vi "应变测试.vi"(15 "stop":bool) -> ()   [LabVIEW 2010]
uses:
  Instance           1 16Saved   应变测试 .vi
  Instance           2 16Saved   应变测试 .vi
  <vilib>/Utility/TradDaqScaling.llb/Convert Strain Gauge Reading (scaler).vi
  <vilib>/Analysis/NI_AALBase.lvlib
panel:
  in  "激 励 电 压":dbl=5.0 format="%.3f"
  in  "应变片灵敏系数":dbl=2.0 format="%.2f"
  in  "置零":bool
  out "电压值\n   (mV)":dbl format="%.2f"
  out "最大挠度\n（mm)":dbl format="%.2f"
  out "电压值 \n   (mV)":dbl format="%.2f"
  out "应变 (με)":cluster{sgl, sgl}(graph)
  out "挠曲轴":cluster{i32[], dbl[]}(graph)
  # "应 变 测 试 实 验"
  # "全   桥"
  # "半   桥"
  # "全桥测试结果"
  # "半桥测试结果"
  # "时间（ms)"
  # "应变值\n（με）"
  # "应变值\n（με）"
  # "挠曲轴"
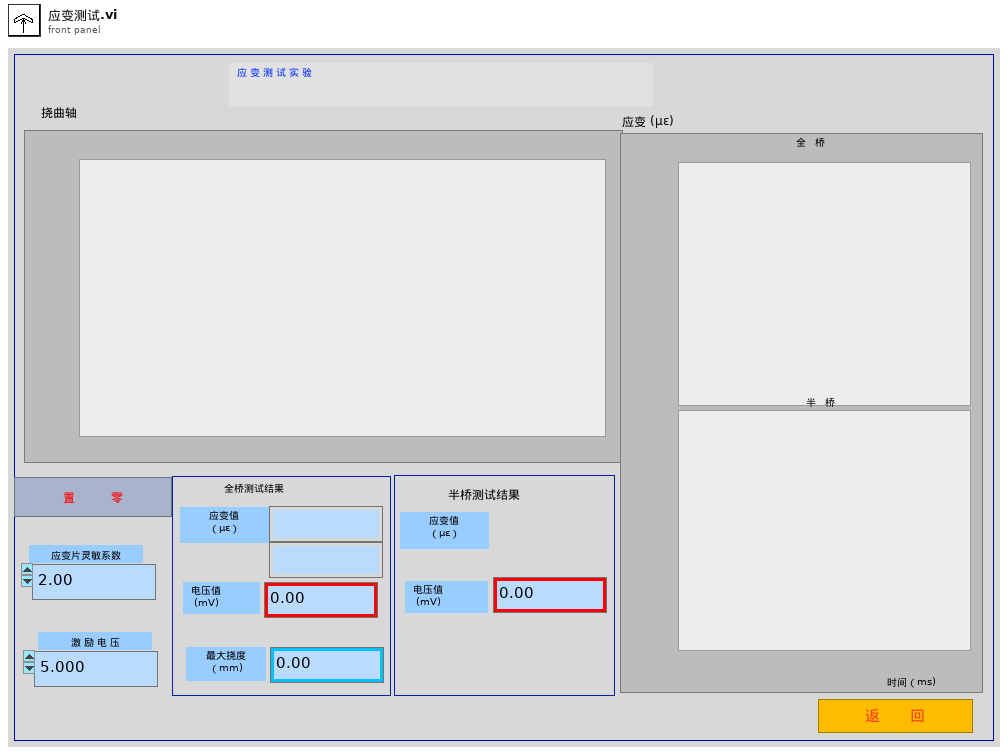
[diagram p1: front panel]
types:
  T1 = cluster{"梁的长度(mm)":dbl, "受力点距固定端(mm)":dbl, "应变片距固定端(mm)":dbl, "梁的厚度(mm)":dbl}
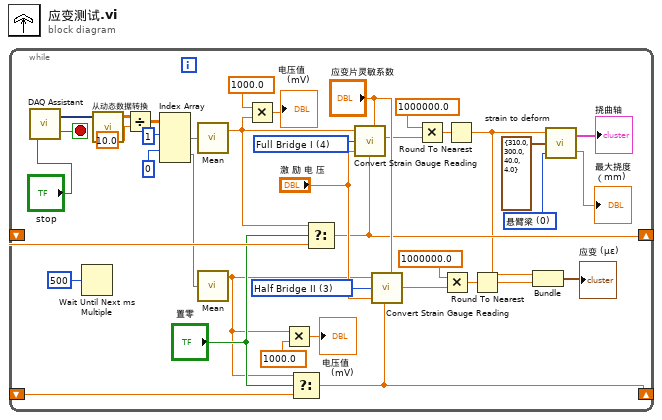
[diagram p0: block diagram]
diagram:
  n1 = while {
    shift-left: _ -> [w39]
    shift-right: [w16] -> _
    shift-right: [w24] -> _
    shift-left: _ -> [w25]
    stop <- w1 stop-if-true
    w9 = u16 0 items=["悬臂梁", "简支梁"] ("梁的结构")
    w34 = u16 3 items=["Qtr Bridge I", "Qtr Bridge II", "Half Bridge I", "Half Bridge II", "Full Bridge I", "Full Bridge II", "Full Bridge III"] ("Bridge Configuration\n(3:Half Bridge II)")
    w35 = u16 4 items=["Qtr Bridge I", "Qtr Bridge II", "Half Bridge I", "Half Bridge II", "Full Bridge I", "Full Bridge II", "Full Bridge III"] ("Bridge Configuration\n(3:Half Bridge II)")
    n2 = call "DAQ Assistant"("stop (F)"="stop") -> ("data"=w20:dynamicdata, "stopped"=w1:bool)  [unwired: 15 in, 2 out]
    n3 = Wait Until Next ms Multiple(millisecond multiple=u32 500 ("毫秒倍数")) -> ()  [unwired: 1 out]
    n4 = call "从动态数据转换"("Dynamic Data Type"=w20) -> ("Array"=w6:dbl[][])  [unwired: 3 in]
    n5 = Divide(x=w6, y=10.0) -> (x/y=w3:dbl[][])
    n6 = Index Array(array=w3, index (row) #1=1 ("disabled index (col)"), index (row) #2=0 ("index (col)")) -> (element #1=w5:dbl[], element #2=w4:dbl[])  [unwired: 2 in]
    n7 = call <vilib>:"Mean.vi"("X"=w5) -> ("mean"=w17:dbl)  [unwired: 1 out]
    n8 = call <vilib>:"Mean.vi"("X"=w4) -> ("mean"=w18:dbl)  [unwired: 1 out]
    n9 = Multiply(x=1000.0, y=w17) -> (x*y=→"电压值\n   (mV)":dbl)
    n10 = Multiply(x=w18, y=1000.0 ("x")) -> (x*y=→"电压值 \n   (mV)":dbl)
    n11 = Select(t=w18, s="置零", f=w25) -> (s? t:f=w24:dbl)
    n12 = Select(t=w17, s="置零", f=w39) -> (s? t:f=w16:dbl)
    n13 = call-poly <vilib>:"Convert Strain Gauge Reading.vi"("Vsg (0.0)"=w17, "Bridge Configuration\n(3:Half Bridge II)"=w35, "Vex (3.33)"="激 励 电 压", "Vinit (0.0)"=w16, "GF (2.0)"="应变片灵敏系数") -> ("Strain"=w23:sgl)  [unwired: 5 in]
    n14 = call-poly <vilib>:"Convert Strain Gauge Reading.vi"("Vsg (0.0)"=w18, "Bridge Configuration\n(3:Half Bridge II)"=w34, "Vex (3.33)"="激 励 电 压", "Vinit (0.0)"=w24, "GF (2.0)"="应变片灵敏系数") -> ("Strain"=w22:sgl)  [unwired: 5 in]
    n15 = Multiply(x=sgl 1000000.0, y=w23) -> (x*y=w37:sgl)
    n16 = Multiply(x=sgl 1000000.0, y=w22) -> (x*y=w31:sgl)
    n17 = Round To Nearest(number=w37) -> (nearest integer value=w11:sgl)
    n18 = Round To Nearest(number=w31) -> (nearest integer value=w21:sgl)
    n19 = Bundle(w11, w21) -> (→"应变 (με)":cluster{sgl, sgl})  [unwired: 1 in]
    n20 = call "strain to deform  .vi"("梁的结构"=w9, "尺寸参数"=T1 {"梁的长度(mm)"=310.0, "受力点距固定端(mm)"=300.0, "应变片距固定端(mm)"=40.0, "梁的厚度(mm)"=4.0}, "Strain"=w11) -> ("max value"=→"最大挠度\n（mm)":dbl, "Deform"=→"挠曲轴":cluster{i32[], dbl[]})
  }
